vi "struct_ads_dw_dT_pT.vi"(8 "Error (Input)":errorcluster, 9 "Temperature in K (Input)":dbl, 10 "Pressure in Pa (Input)":dbl, 11 "Reference working pair (Input)":i64) -> (0 "Error (Output)":errorcluster caption="Error(Output)", 3 "Der. of loading wrt. temperature in kg/kg/K (Output)":dbl)   [LabVIEW 2017]
doc: "ads_dw_dT_pT:\n * -------------\n *\n * Calculates derivative of equilibrium loading w with respect to temperature\n * T in kg/kg/K depending on equilibrium pressure p in Pa and equilibrium\n * temperature T in K.\n *\n * Parameters:\n * -----------\n * double p_Pa:\n * Equilibrium pressure in Pa.\n * double T_K:\n * Equilibrium temperature in K.\n * struct *WorkingPair:\n * Pointer of WorkingPair-struct.\n *\n * Returns:\n * --------\n * double:\n * Derivative of equilibrium loading wrt. temperature in kg/kg/K.\n *\n * History:\n * --------\n * 07/13/2021, by Jannik Driesel (supervised by Mirko Engelpracht):\n * First implementation."
uses:
  data/win32bit/libsorpPropLib.dll
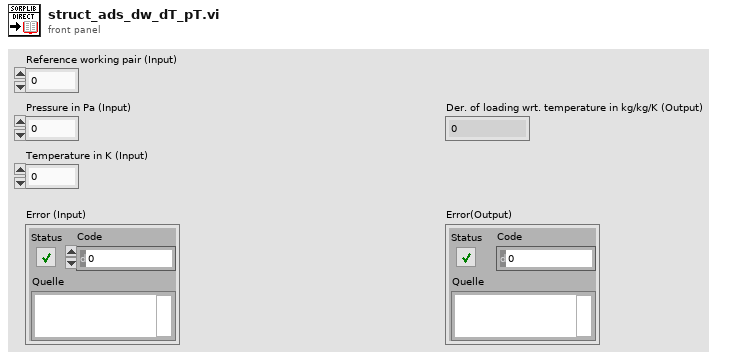
[diagram p1: front panel]
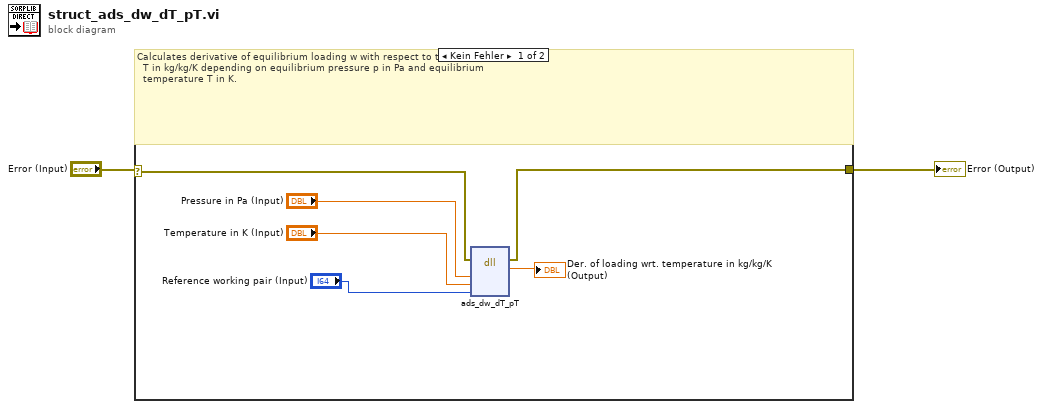
[diagram p0: block diagram]
diagram:
  n1 = case shown="Kein Fehler" "Error (Input)" {
    selector: "Error (Input)" -> [w5 w9]
    tunnel: [w4 w9] -> w1
    frame No Error {
      # "Calculates derivative of equilibrium loading w with respect to temperature\n  T in kg/kg/K depending on equilibrium pressure p in Pa and equilibrium\n  temperature T in K."
      n2 = dll-call lib="D:/Driesel/SorpLibLocal/LabVIEW_wrapper/data/win32bit/libsorpPropLib.dll" fn="ads_dw_dT_pT"(error in=w5, "p_Pa"="Pressure in Pa (Input)", "T_K"="Temperature in K (Input)", "workingPair"="Reference working pair (Input)") -> (error out=w4:errorcluster, "dw_dT_kgkgK"=→"Der. of loading wrt. temperature in kg/kg/K (Output)":dbl)  [unwired: 5 in, 1 out]
    }
    frame Error {
      # "Error - No calculations"
    }
  }
  "Error (Output)" <- w1
